vi "CalcChannelWidth_HH.vi"(1 "HH binning":u16, 2 "channel count":i32, 3 "rebinning":u16) -> (0 "channel width (ns)":dbl format="%.6f")   [LabVIEW 2009]
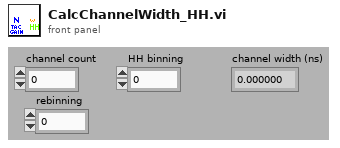
[diagram p1: front panel]
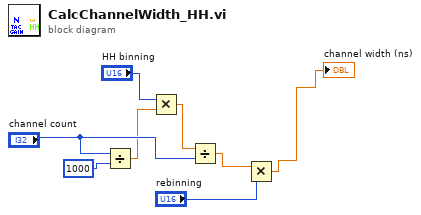
[diagram p0: block diagram]
diagram:
  n1 = Divide(x="channel count", y=1000) -> (x/y=w5:dbl)
  n2 = Multiply(x="HH binning", y=w5) -> (x*y=w4:dbl)
  n3 = Divide(x=w4, y="channel count") -> (x/y=w3:dbl)
  n4 = Multiply(x=w3, y="rebinning") -> (x*y=→"channel width (ns)":dbl)
